vi "Render Captain.vi"(7 "Renderer":refnum<class "Renderer.lvclass">, 8 "error in (no error)":errorcluster, 11 "Ship in":refnum<class "Ship.lvclass">) -> (0 "error out":errorcluster)   [LabVIEW 2021, in "Ship.lvclass"]
uses:
  Ship.lvclass
  Renderer/Renderer.lvclass
  Ship.lvclass/Ship.ctl
  Re-use Libraries/Vector 2D/Vector 2D.lvclass
  LabSDL2/Source/Libraries/SDL2 Utility/Point (I32).ctl
  LabSDL2/Source/Libraries/SDL2 Utility/SDL2 Utility.lvlib
  Control State/Control State.lvclass
  Resource Manager/Resource Manager.lvclass
  Element/Element.lvclass
  Math/Math.lvlib
panel:
  in  "y":T1={"x"=-17, "y"=-300}
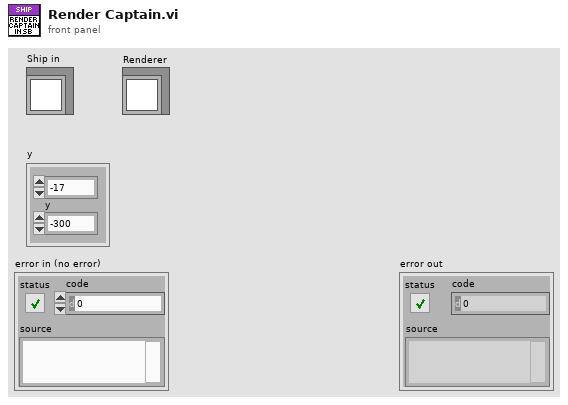
[diagram p1: front panel]
types:
  T1 = typedef "SDL2 Utility.lvlib/Point (I32).ctl" = cluster{"x":i32, "y":i32}
  T2 = typedef "Constants.ctl" = cluster{"Colours":cluster{"OK":u32, "Warning":u32, "Error":u32, "Red":u32, "Green":u32, "Blue":u32, "Yellow":u32}, "System":cluster{"Target Frames Second":dbl, "World Size":T1, "Window Size":T1, "Battle Area Size":T1, "Sidebar Scaling":sgl, "Sidebar Width":i32, "SC2 Frame Rate [Seconds/Frame]":sgl}, "Game":cluster{"Maximum Asteroids":i32, "Max Energy":i32, "Max Crew":i32, "Maximum Stars":i32}}
  T3 = typedef "Element.lvclass/Player Type.ctl" = enum16{"Neutral", "Player 1", "Player 2"}
  T4 = typedef "Control State.lvclass/Button State.ctl" = enum16{"Undefined", "Pressed", "Released", "Held", "Not Held"}
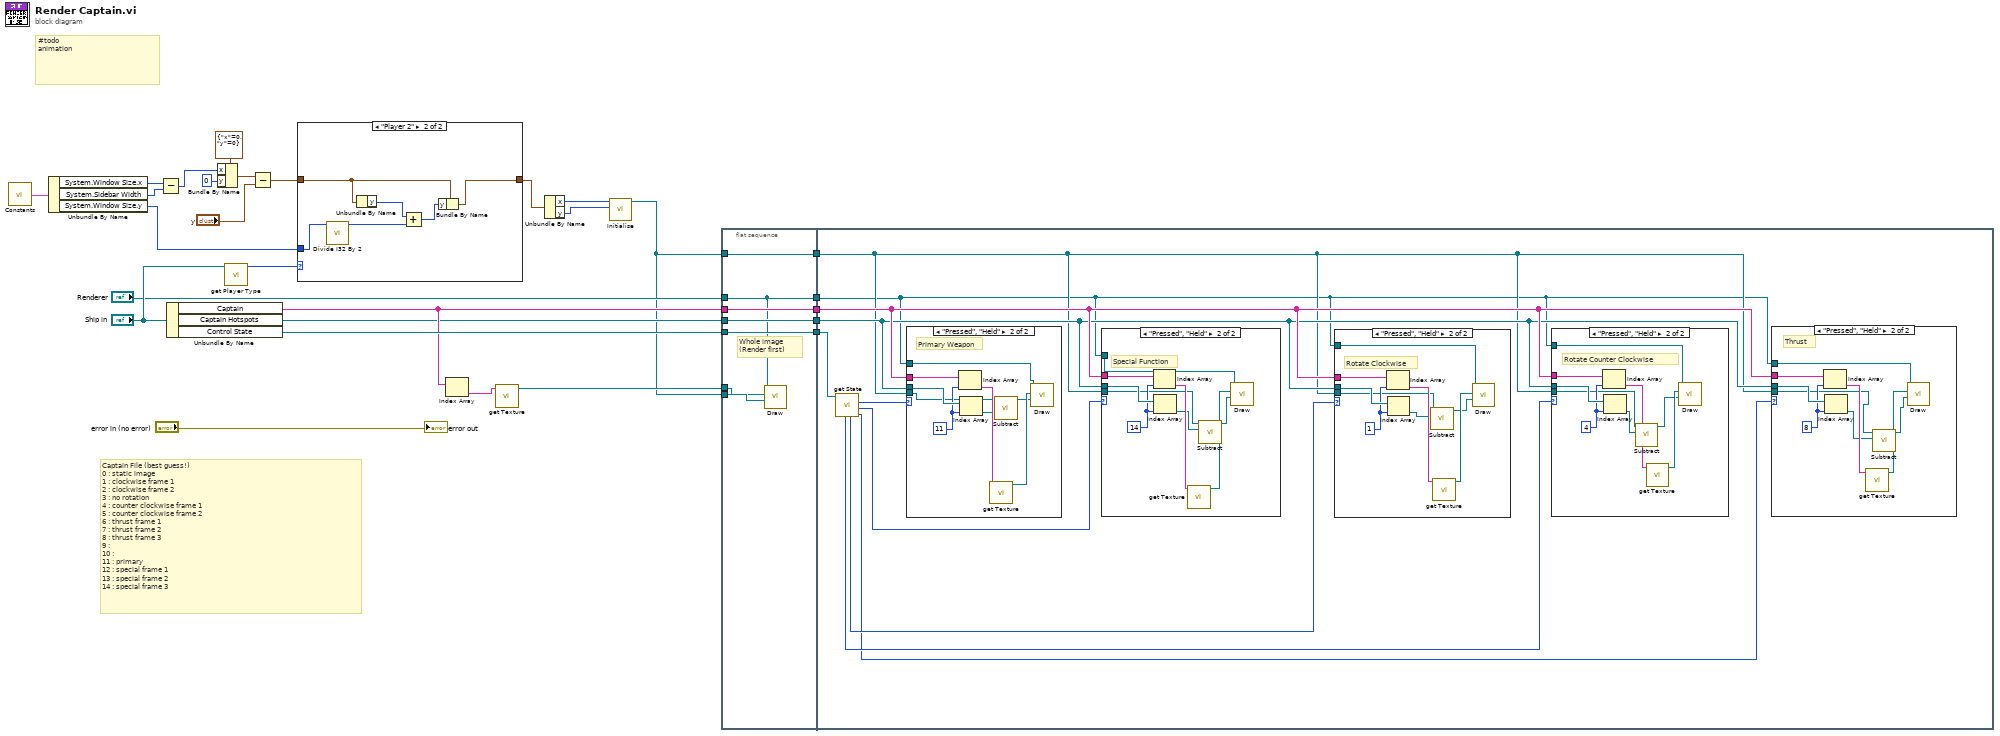
[diagram p0: block diagram]
diagram:
  # "Captain File (best guess!)\n0 : static image\n1 : clockwise frame 1\n2 : clockwise frame 2\n3 : no rotation\n4 : counter clockwise frame 1\n5 : counter clockwise frame 2\n6 : thrust frame 1\n7 : thrust frame 2\n8 : thrust frame 3\n9 :\n10 :\n11 : primary\n12 : special frame 1\n13 : special frame 2\n14 : special frame 3"
  # "#todo\nanimation"
  n1 = call "Constants.vi"() -> ("Constants"=w24:T2)
  n2 = Unbundle By Name(w24) -> ("System.Window Size.x"=w22:i32, "System.Sidebar Width"=w21:i32, "System.Window Size.y"=w16:i32)
  n3 = Subtract(x=w22, y=w21) -> (x-y=w20:i32)
  n4 = Unbundle By Name("Ship in") -> ("Captain"=w27:string[], "Captain Hotspots"=w26:refnum<class "Vector 2D.lvclass">[], "Control State"=w28:refnum<class "Control State.lvclass">)
  n5 = Bundle By Name(cluster=T1 {"x"=0, "y"=0} ("Icon Offsets"), "x"=w20, "y"=0) -> (w19:T1)
  n6 = call "get Player Type.vi"("Element in"="Ship in") -> ("Player Type"=w13:T3)  [unwired: 10 in]
  n7 = Subtract(x=w19, y="y") -> (x-y=w17:T1)
  n8 = case shown="\"Player 2\"" w13 {
    tunnel: [w29 w32] -> w2
    tunnel: w17 -> [w29 w33]
    tunnel: w16 -> [_ w31]
    frame "Player 1", Default {
    }
    frame "Player 2" {
      n9 = call "Divide I32 By 2.vi"("Value"=w31) -> ("Value/2"=w30:i32)  [unwired: 10 in]
      n10 = Unbundle By Name(w33) -> ("y"=w34:i32)
      n11 = Add(x=w34, y=w30) -> (x+y=w35:i32)
      n12 = Bundle By Name(cluster=w33, "y"=w35) -> (w32:T1)
    }
  }
  n13 = Index Array(array=w27) -> (element=w15:string)  [unwired: 1 in]
  n14 = call "get Texture.vi"("Texture Name"=w15) -> ("Texture"=w8:refnum<class "Texture.lvclass">)  [unwired: 10 in]
  n15 = Unbundle By Name(w2) -> ("x"=w4:i32, "y"=w3:i32)
  n16 = call "Initialise.vi"("y"=w3, "x"=w4) -> ("Vector 2D out"=w1:refnum<class "Vector 2D.lvclass">)  [unwired: 9 in]
  n17 = flat-sequence {
    tunnel: w1 -> [w39]
    tunnel: w26 -> [w40]
    tunnel: w27 -> [w41]
    tunnel: w28 -> [w42]
    tunnel: [w42] -> w12
    tunnel: [w41] -> w11
    tunnel: [w40] -> w10
    tunnel: [w39] -> w9
    tunnel: w1 -> [w38]
    tunnel: w8 -> [w37]
    tunnel: "Renderer" -> [w36]
    tunnel: [w36] -> w6
    tunnel: w12 -> [w52]
    tunnel: w11 -> [w46]
    tunnel: w10 -> [w45]
    tunnel: w9 -> [w44]
    tunnel: w6 -> [w43]
    frame #0 {
      # "Whole image\n(Render first)"
      n18 = call "Draw.vi"("Destination"=w38, "Texture"=w37, "Renderer"=w36) -> ()  [unwired: 8 in, 1 out]
    }
    frame #1 {
      n19 = call "get State.vi"("Control State in"=w52) -> ("Thrust"=w47:T4, "Special Function"=w50:T4, "Primary Weapon"=w51:T4, "Rotate Clockwise"=w49:T4, "Rotate Counter Clockwise"=w48:T4)  [unwired: 6 in]
      n20 = case shown="\"Pressed\", \"Held\"" w51 {
        tunnel: w46 -> [_ w97]
        tunnel: w45 -> [_ w96]
        tunnel: w44 -> [_ w90]
        tunnel: w43 -> [_ w91]
        frame Default {
        }
        frame "Pressed", "Held" {
          w95 = 11 ("index")
          # "Primary Weapon"
          n21 = Index Array(array=w97, index=w95) -> (element=w93:string)
          n22 = Index Array(array=w96, index=w95) -> (element=w89:refnum<class "Vector 2D.lvclass">)
          n23 = call "get Texture.vi"("Texture Name"=w93) -> ("Texture"=w94:refnum<class "Texture.lvclass">)  [unwired: 10 in]
          n24 = call "Subtract.vi"("B"=w89, "A"=w90) -> ("A-B"=w92:refnum<class "Vector 2D.lvclass">)  [unwired: 9 in]
          n25 = call "Draw.vi"("Destination"=w92, "Texture"=w94, "Renderer"=w91) -> ()  [unwired: 8 in, 1 out]
        }
      }
      n26 = case shown="\"Pressed\", \"Held\"" w50 {
        tunnel: w46 -> [_ w88]
        tunnel: w45 -> [_ w87]
        tunnel: w44 -> [_ w81]
        tunnel: w43 -> [_ w83]
        frame Default {
        }
        frame "Pressed", "Held" {
          w86 = 14 ("index")
          # "Special Function"
          n27 = Index Array(array=w88, index=w86) -> (element=w84:string)
          n28 = Index Array(array=w87, index=w86) -> (element=w80:refnum<class "Vector 2D.lvclass">)
          n29 = call "get Texture.vi"("Texture Name"=w84) -> ("Texture"=w85:refnum<class "Texture.lvclass">)  [unwired: 10 in]
          n30 = call "Subtract.vi"("B"=w80, "A"=w81) -> ("A-B"=w82:refnum<class "Vector 2D.lvclass">)  [unwired: 9 in]
          n31 = call "Draw.vi"("Destination"=w82, "Texture"=w85, "Renderer"=w83) -> ()  [unwired: 8 in, 1 out]
        }
      }
      n32 = case shown="\"Pressed\", \"Held\"" w49 {
        tunnel: w46 -> [_ w79]
        tunnel: w45 -> [_ w78]
        tunnel: w44 -> [_ w72]
        tunnel: w43 -> [_ w74]
        frame Default {
        }
        frame "Pressed", "Held" {
          w77 = 1 ("index")
          # "Rotate Clockwise"
          n33 = Index Array(array=w79, index=w77) -> (element=w75:string)
          n34 = Index Array(array=w78, index=w77) -> (element=w71:refnum<class "Vector 2D.lvclass">)
          n35 = call "Subtract.vi"("B"=w71, "A"=w72) -> ("A-B"=w73:refnum<class "Vector 2D.lvclass">)  [unwired: 9 in]
          n36 = call "get Texture.vi"("Texture Name"=w75) -> ("Texture"=w76:refnum<class "Texture.lvclass">)  [unwired: 10 in]
          n37 = call "Draw.vi"("Destination"=w73, "Texture"=w76, "Renderer"=w74) -> ()  [unwired: 8 in, 1 out]
        }
      }
      n38 = case shown="\"Pressed\", \"Held\"" w48 {
        tunnel: w46 -> [_ w70]
        tunnel: w45 -> [_ w69]
        tunnel: w44 -> [_ w63]
        tunnel: w43 -> [_ w65]
        frame Default {
        }
        frame "Pressed", "Held" {
          w68 = 4 ("index")
          # "Rotate Counter Clockwise"
          n39 = Index Array(array=w70, index=w68) -> (element=w66:string)
          n40 = Index Array(array=w69, index=w68) -> (element=w62:refnum<class "Vector 2D.lvclass">)
          n41 = call "Subtract.vi"("B"=w62, "A"=w63) -> ("A-B"=w64:refnum<class "Vector 2D.lvclass">)  [unwired: 9 in]
          n42 = call "get Texture.vi"("Texture Name"=w66) -> ("Texture"=w67:refnum<class "Texture.lvclass">)  [unwired: 10 in]
          n43 = call "Draw.vi"("Destination"=w64, "Texture"=w67, "Renderer"=w65) -> ()  [unwired: 8 in, 1 out]
        }
      }
      n44 = case shown="\"Pressed\", \"Held\"" w47 {
        tunnel: w46 -> [_ w61]
        tunnel: w45 -> [_ w60]
        tunnel: w44 -> [_ w54]
        tunnel: w43 -> [_ w56]
        frame Default {
        }
        frame "Pressed", "Held" {
          w59 = 8 ("index")
          # "Thrust"
          n45 = Index Array(array=w61, index=w59) -> (element=w57:string)
          n46 = Index Array(array=w60, index=w59) -> (element=w53:refnum<class "Vector 2D.lvclass">)
          n47 = call "get Texture.vi"("Texture Name"=w57) -> ("Texture"=w58:refnum<class "Texture.lvclass">)  [unwired: 10 in]
          n48 = call "Subtract.vi"("B"=w53, "A"=w54) -> ("A-B"=w55:refnum<class "Vector 2D.lvclass">)  [unwired: 9 in]
          n49 = call "Draw.vi"("Destination"=w55, "Texture"=w58, "Renderer"=w56) -> ()  [unwired: 8 in, 1 out]
        }
      }
    }
  }
  "error out" <- "error in (no error)"
